vi "Initialize Data Acquisition.vi"(8 "error in (no error)":errorcluster, 11 "Hardware Resources in":T1={"State"=enum."Idle S3DK", "Settings"="", "Status"={"Online"=FALSE, "Buffer"=FALSE, "Config"=FALSE, "Connect"=FALSE}, "S3DK"={"Signals"={"Phasor"=[], "Analog"=[], "Digital"=[]}}, "Tick"=0}) -> (0 "error out":errorcluster, 3 "Hardware Resources out":T1={"State"=enum."Idle S3DK", "Settings"="", "Status"={"Online"=FALSE, "Buffer"=FALSE, "Config"=FALSE, "Connect"=FALSE}, "S3DK"={"Signals"={"Phasor"=[], "Analog"=[], "Digital"=[]}}, "Tick"=0})   [LabVIEW 2017, in "Acquisition.lvlib"]
doc: "Initialize the hardware references."
uses:
  Acquisition.lvlib
  Acquisition Settings.ctl
  Acquisition State.ctl
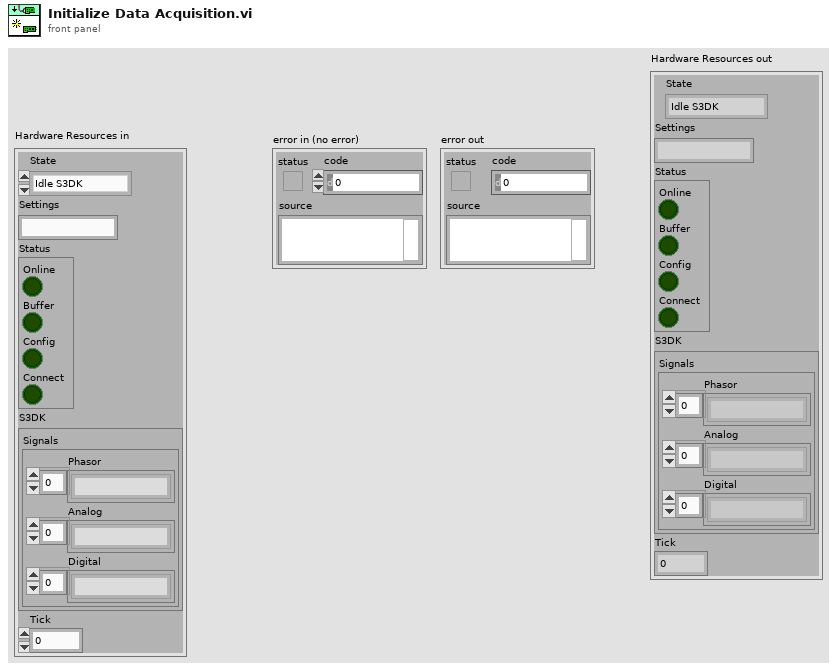
[diagram p1: front panel]
types:
  T1 = typedef "Acquisition.lvlib/Acquisition Settings.ctl" = cluster{"State":T2, "Settings":string, "Status":cluster{"Online":bool, "Buffer":bool, "Config":bool, "Connect":bool}, "S3DK":cluster{"Signals":cluster{"Phasor":string[], "Analog":string[], "Digital":string[]}}, "Tick":u32}
  T2 = typedef "Acquisition.lvlib/Acquisition State.ctl" = enum16{"Idle", "Idle S3DK", "Acquiring S3DK", "Idle CSV", "Acquiring CSV"}
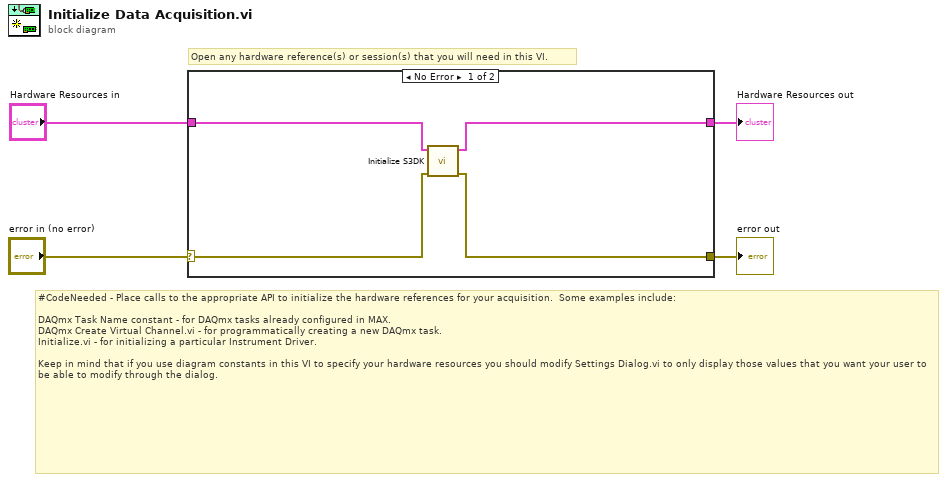
[diagram p0: block diagram]
diagram:
  # "Open any hardware reference(s) or session(s) that you will need in this VI."
  # "#CodeNeeded - Place calls to the appropriate API to initialize the hardware references for your acquisition.  Some examples include:\n\nDAQmx Task Name constant - for DAQmx tasks already configured in MAX.\nDAQmx Create Virtual Channel.vi - for programmatically creating a new DAQmx task.\nInitialize.vi - for initializing a particular Instrument Driver.\n\nKeep in mind that if you use diagram constants in this VI to specify your hardware resources you should modify Settings Dialog.vi to only display those values that you want your user to be able to modify through the dialog."
  n1 = case shown="No Error" "error in (no error)" {
    selector: "error in (no error)" -> [w6 w9]
    tunnel: [w5 w9] -> w3
    tunnel: "Hardware Resources in" -> [w8 w10]
    tunnel: [w7 w10] -> w1
    frame No Error {
      n2 = call "Initialize S3DK.vi"("error in (no error)"=w6, "Settings IN"=w8) -> ("error out"=w5:errorcluster, "Settings OUT"=w7:T1)  [unwired: 8 in]
    }
    frame Error {
    }
  }
  "Hardware Resources out" <- w1
  "error out" <- w3
